vi "SetSpeedProperties.vi"(8 "OpState":string, 9 "data":T2, 10 "data event properties in":T1[](array[typedef])) -> (2 "data event properties out":T1[](array[typedef]))   [LabVIEW 2017, in "McsaDataEventCreator.lvlib"]
uses:
  <vilib>/addons/InsightCM/Devices/Shared/Mcsa/McsaDataEventCreator/McsaDataEventCreator.lvlib
  <vilib>/addons/InsightCM/MessageBus/Base/controls/KeyValuePair.ctl
  <vilib>/addons/InsightCM/Devices/Shared/Common/DataFlow/controls/Data.ctl
  <vilib>/addons/InsightCM/Utilities/DataAccessors/controls/wfmSGL_DVR.ctl
  <vilib>/addons/PointValueMap/controls/PointMap.ctl
  <vilib>/addons/InsightCM/Devices/Shared/Common/DataFlow/controls/Type.ctl
  <vilib>/addons/PointValueMap/PointValueMap.lvlib
  <vilib>/addons/InsightCM/Utilities/PropertyHelpers/PropertyHelpers.lvlib
  <vilib>/addons/InsightCM/Devices/Shared/Common/DataFlow/DataFlow.lvlib
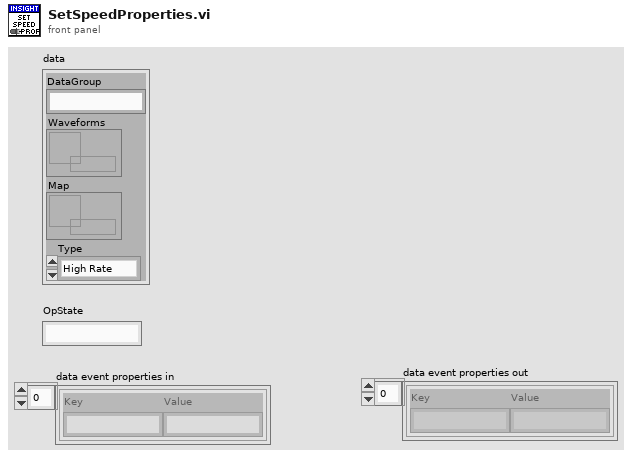
[diagram p1: front panel]
types:
  T1 = typedef "KeyValuePair.ctl" = cluster{"Key":string, "Value":string}
  T2 = typedef "DataFlow.lvlib/Data.ctl" = cluster{"DataGroup":string, "Waveforms":T3, "Map":T4, "Type":T5}
  T3 = typedef "wfmSGL_DVR.ctl" = refnum<data-value>
  T4 = typedef "PointValueMap.lvlib/PointMap.ctl" = refnum<data-value>
  T5 = typedef "DataFlow.lvlib/Type.ctl" = enum16{"High Rate", "Low Rate", "Burst Mode"}
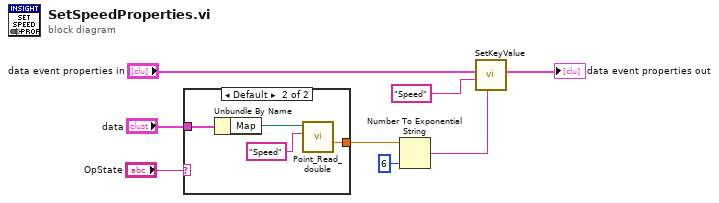
[diagram p0: block diagram]
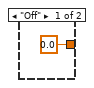
[diagram p2: hidden frame]
diagram:
  n1 = case shown="Default" "OpState" {
    tunnel: "data" -> [_ w13]
    tunnel: [0.0 ("Value") w10] -> w3
    frame "Off" {
    }
    frame Default {
      n2 = Unbundle By Name(w13) -> ("Map"=w11:T4)
      n3 = call <vilib>:"Point_Read_double.vi"("Tag"="Speed", "Map"=w11) -> ("Value"=w10:dbl)  [unwired: 4 in, 5 out]
    }
  }
  n4 = Number To Exponential String(number=w3, precision (6)=i16 6) -> (E-format string=w2:string)  [unwired: 2 in]
  n5 = call <vilib>:"SetKeyValue.vi"("value"=w2, "key"="Speed", "key value pairs"="data event properties in") -> ("key value pairs out"=→"data event properties out":T1[])  [unwired: 8 in]
